vi "DIAdem Run Automation Command.vi"(8 "error in (no error)":errorcluster, 9 "asynchronous? (F)":bool, 10 "command":string, 11 "DIAdem Reference":T1) -> (0 "error out":errorcluster, 3 "DIAdem Reference":T1)   [LabVIEW 2020]
doc: "This VI sends a command directly to the DIAdem environment. You can use this VI to call any of the DIAdem internal functions."
uses:
  <vilib>/ExportToExcel/DIAdem Reference.ctl
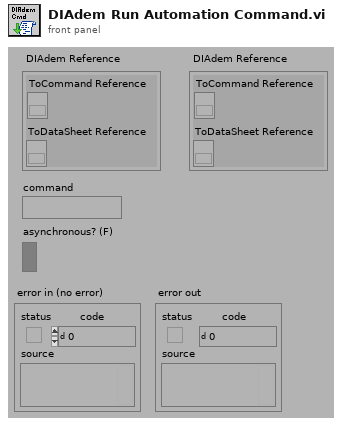
[diagram p1: front panel]
types:
  T1 = typedef "DIAdem Reference.ctl" = cluster{"ToCommand Reference":refnum<k7>, "ToDataSheet Reference":refnum<k7>}
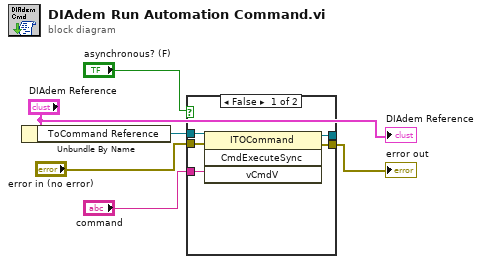
[diagram p0: block diagram]
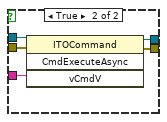
[diagram p2: hidden frame]
diagram:
  n1 = Unbundle By Name("DIAdem Reference") -> ("ToCommand Reference"=w4:refnum<k7>)
  n2 = case shown="False" "asynchronous? (F)" {
    tunnel: [w11 w16] -> _
    tunnel: w4 -> [w10 w15]
    tunnel: [w9 w14] -> w1
    tunnel: "command" -> [w8 w13]
    tunnel: "error in (no error)" -> [w7 w12]
    frame False {
      n3 = invoke class="ITOCommand" method="CmdExecuteSync"(reference=w10, error in=w7, "vCmdV"=w8) -> (reference out=w11:refnum<k7>, error out=w9:errorcluster)  [unwired: 1 in, 2 out]
    }
    frame True {
      n4 = invoke class="ITOCommand" method="CmdExecuteAsync"(reference=w15, error in=w12, "vCmdV"=w13) -> (reference out=w16:refnum<k7>, error out=w14:errorcluster)  [unwired: 1 in, 2 out]
    }
  }
  "error out" <- w1
  "DIAdem Reference" <- "DIAdem Reference"
